vi "Write to pump 2.vi"(8 "error in (no error)":errorcluster, 9 "Write wait between \ncharacters (default 10 ms)":i32=10, 10 "String to write":string="\r", 11 "VISA resource name":refnum<visa-resource-name>="COM3") -> (0 "error out":errorcluster, 3 "VISA resource name out":refnum<visa-resource-name>)   [LabVIEW 2016]
uses:
  <vilib>/Instr/_visa.llb/VISA Configure Serial Port (Instr).vi
panel:
  # "Author: Barbara Stekas\nDate: 6/29/2015 \n\nConfigures connection and writes a string + termination character (cr) to\nthe VISA resource input. String is sent one letter at a time with a wait between\nletters given by \"Write wait.\" 10 ms is the fastest it seems the Harvard PHD 2000 \npump can handle. Closes VISA session at end."
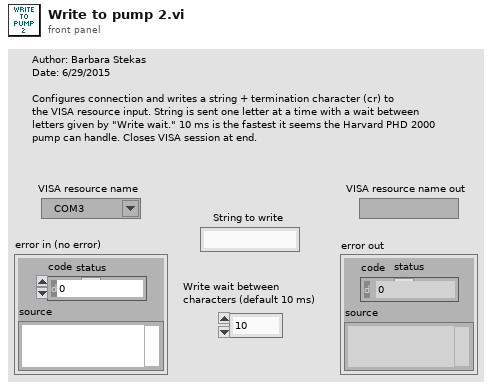
[diagram p1: front panel]
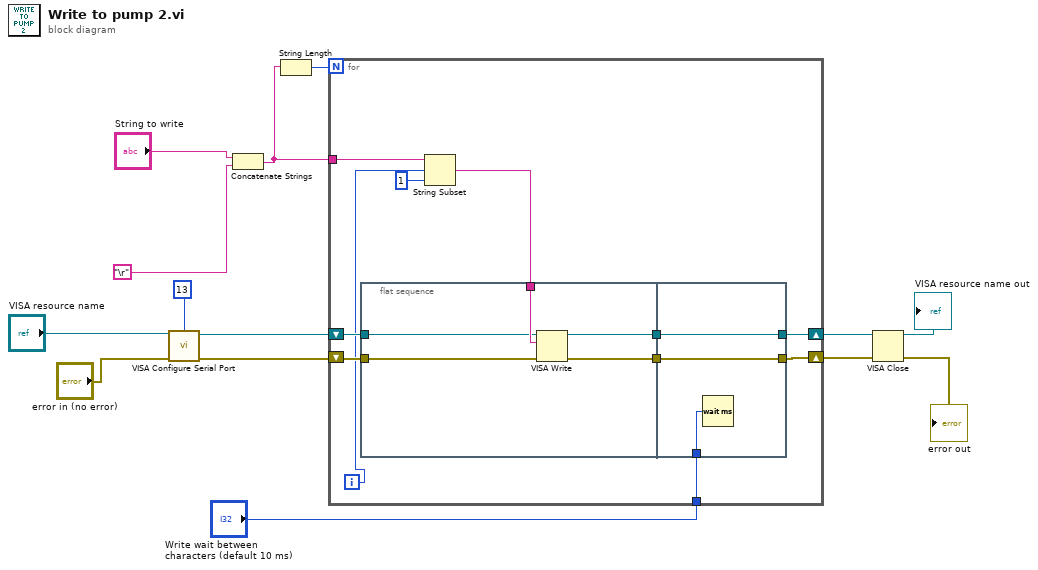
[diagram p0: block diagram]
diagram:
  n1 = call-poly "VISA Configure Serial Port"("VISA resource name"="VISA resource name", "termination char\n(0xA = '\\n' = LF)"=u8 13 ("termination char\n(0xA = '\\n' = LF)"), "error in (no error)"="error in (no error)") -> ("VISA resource name out"=w7:refnum<visa-resource-name>, "error out"=w8:errorcluster)  [unwired: 11 in]
  n2 = Concatenate Strings("String to write", "\r") -> (w4:string)
  n3 = String Length(string=w4) -> (length=w5:i32)
  n4 = for {
    N: w5 -> [_]
    tunnel: "Write wait between \ncharacters (default 10 ms)" -> [w21]
    tunnel: w4 -> [w16]
    shift-right: [w18] -> w10
    shift-left: w7 -> [w19]
    shift-right: [w17] -> w11
    shift-left: w8 -> [w20]
    i -> [w15]
    n5 = flat-sequence {
      tunnel: [w28] -> w23
      tunnel: [w27] -> w22
      tunnel: w13 -> [w26]
      tunnel: w20 -> [w24]
      tunnel: w19 -> [w25]
      tunnel: [w30] -> w17
      tunnel: [w31] -> w18
      tunnel: w23 -> [w31]
      tunnel: w22 -> [w30]
      tunnel: w21 -> [w29]
      frame #0 {
        n6 = VISA Write(VISA resource name=w25, write buffer=w26, error in (no error)=w24) -> (VISA resource name out=w28:refnum<visa-resource-name>, error out=w27:errorcluster)  [unwired: 1 out]
      }
      frame #1 {
        n7 = Wait (ms)(milliseconds to wait=w29) -> ()  [unwired: 1 out]
      }
    }
    n8 = String Subset(string=w16, offset (0)=w15, length (rest)=1 ("length (rest)")) -> (substring=w13:string)
  }
  "error out" <- w11
  "VISA resource name out" <- w10
  n9 = VISA Close(VISA resource name=w10, error in (no error)=w11) -> ()  [unwired: 1 out]
